vi "TriggerSetup_CreateGalvoTask.vi"(7 "Scanrate (pixels/s)":u32(ring)=10000 items=["250 kHz"=250000, "125 kHz"=125000, "50 kHz (!)"=50000, "25 kHz (!)"=25000, "10 kHz (?)"=10000, "5 kHz (?)"=5000, "2 kHz"=2000, "1 kHz"=1000, "500 Hz"=500, "200 Hz"=200, "100 Hz"=100], 8 "error in":errorcluster, 9 "physical channel ao0":tag="Dev1/ao0", 10 "physical channel ao1":tag="Dev1/ao1", 11 "Scanning waveforms":dbl[][](array[numeric])) -> (0 "error out":errorcluster, 3 "write task":refnum<k21>, 4 "Length (scanning waveforms)":i32)   [LabVIEW 2020]
uses:
  <vilib>/DAQmx/create/channels.llb/DAQmx Create Channel (AO-Voltage-Basic).vi
  <vilib>/DAQmx/configure/timing.llb/DAQmx Timing (Sample Clock).vi
  <vilib>/DAQmx/configure/trigger.llb/DAQmx Start Trigger (Digital Edge).vi
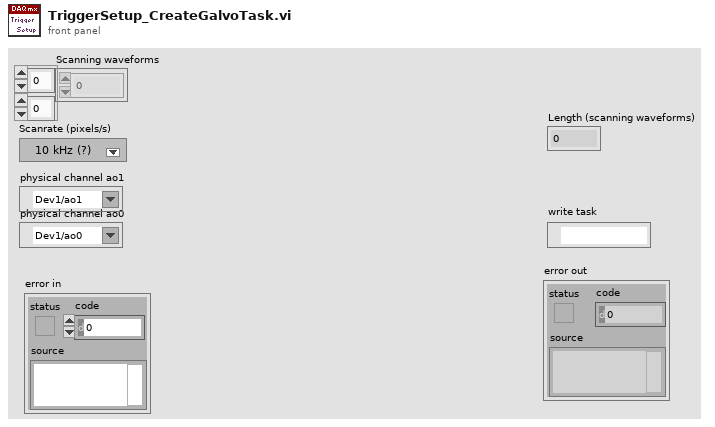
[diagram p1: front panel]
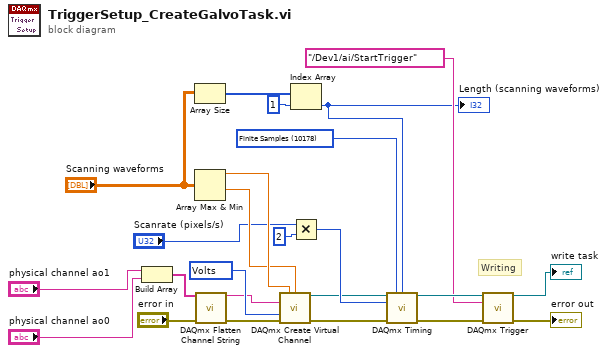
[diagram p0: block diagram]
diagram:
  w13 = 10178 items=["Finite Samples"=10178, "Continuous Samples"=10123, "Hardware Timed Single Point"=12522] ("sample mode")
  w24 = 10348 items=["Volts"=10348, "From Custom Scale"=10065] ("units")
  # "Writing"
  n1 = Build Array("physical channel ao1", "physical channel ao0") -> (w22:tag[])
  n2 = Array Size(array="Scanning waveforms") -> (size(s)=w17:i32[])
  n3 = Array Max & Min(array="Scanning waveforms") -> (max value=w21:dbl, min value=w20:dbl)  [unwired: 2 out]
  n4 = call <vilib>:"DAQmx Flatten Channel String.vi"("names in"=w22, "error in"="error in") -> ("names out"=w19:string, "error out"=w23:errorcluster)  [unwired: 12 in]
  n5 = call-poly <vilib>:"DAQmx Create Virtual Channel.vi"("maximum value"=w21, "minimum value"=w20, "physical channels"=w19, "units"=w24, "error in"=w23) -> ("task out"=w3:refnum<k21>, "error out"=w4:errorcluster)  [unwired: 9 in]
  n6 = Index Array(array=w17, index=1) -> (element=w7:i32)
  "Length (scanning waveforms)" <- w7
  n7 = Multiply(x="Scanrate (pixels/s)", y=u32 2) -> (x*y=w12:u32)
  n8 = call-poly <vilib>:"DAQmx Timing.vi"("task/channels in"=w3, "sample mode"=w13, "samples per channel"=w7, "rate"=w12, "error in"=w4) -> ("task out"=w15:refnum<k21>, "error out"=w14:errorcluster)  [unwired: 9 in]
  n9 = call-poly <vilib>:"DAQmx Trigger.vi"("task/channels in"=w15, "source"=tag "/Dev1/ai/StartTrigger", "error in"=w14) -> ("task out"=→"write task":refnum<k21>, "error out"=→"error out":errorcluster)  [unwired: 11 in]
